vi "New Task Setting Editor.vi"(7 "Task Setting Editor in":refnum<class "Task Setting Editor.lvclass">, 8 "error in (no error)":errorcluster) -> (0 "error out":errorcluster, 3 "Task Setting Editor out":refnum<class "Task Setting Editor.lvclass">)   [LabVIEW 2017, in "Task Setting Editor.lvlib" / "Task Setting Editor.lvclass"]
uses:
  Task Setting Editor.lvclass
  BuildWorker/Classes/Task/Task.lvclass
  Task Setting Editor.lvclass/Task Setting Editor.ctl
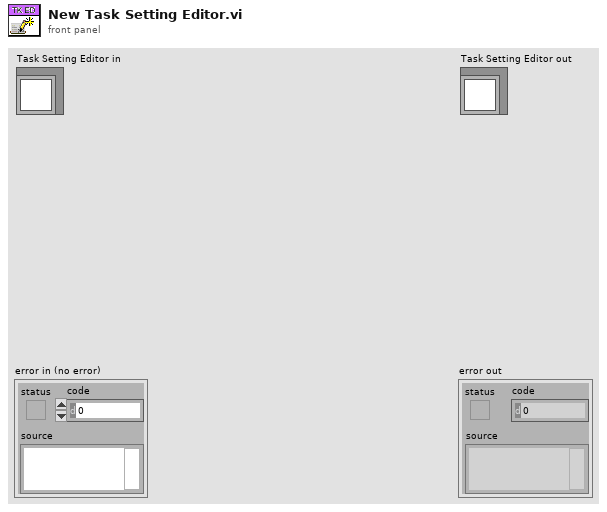
[diagram p1: front panel]
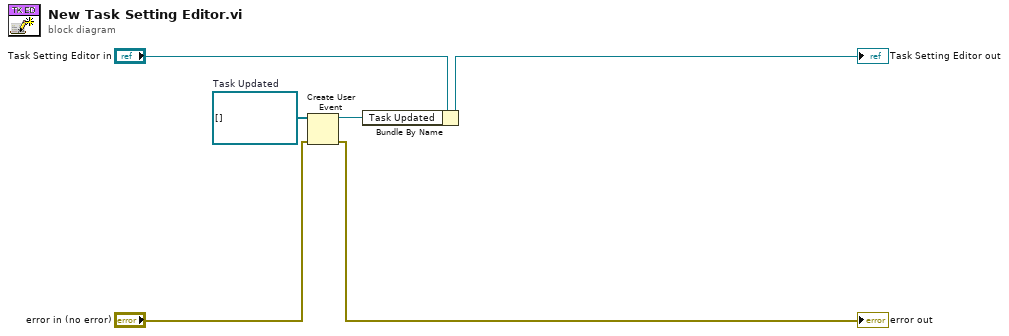
[diagram p0: block diagram]
diagram:
  w5 = refnum<class "Task.lvclass">[] []  # Task Updated
  n1 = Create User Event(user event datatype=w5, error in="error in (no error)") -> (user event=w3:refnum<user-event>, error out=→"error out":errorcluster)
  n2 = Bundle By Name(cluster="Task Setting Editor in", "Task Updated"=w3) -> (→"Task Setting Editor out":refnum<class "Task Setting Editor.lvclass">)
